vi "ROI ID to ROI enum.vi"(6 "ROI ID":i32) -> (2 "ROI Enum":T1)   [LabVIEW 2020]
uses:
  Typedefs/ROI ID Enum.ctl
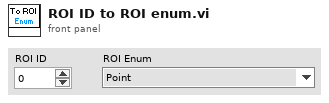
[diagram p1: front panel]
types:
  T1 = typedef "ROI ID Enum.ctl" = enum16{"Point", "MiniScan", "Comp. MiniScan", "Rectangle", "Comp. volume", "Arb. plane point", "None"}
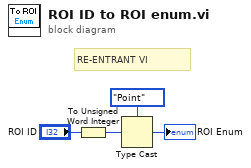
[diagram p0: block diagram]
diagram:
  # "RE-ENTRANT VI"
  n1 = To Unsigned Word Integer(number="ROI ID") -> (unsigned 16bit integer=w3:u16)
  n2 = Type Cast(type=ROI_ID_Enum."Point" ("ROI Enum"), x=w3) -> (*(type *) &x=→"ROI Enum":T1)
